vi "START1.vi"() -> ()   [LabVIEW 2024]
uses:
  <vilib>/Utility/file.llb/Read Delimited Spreadsheet (DBL).vi
panel:
  in  "stop":bool
  out "Flow Rate Display":dynamicdata(graph)
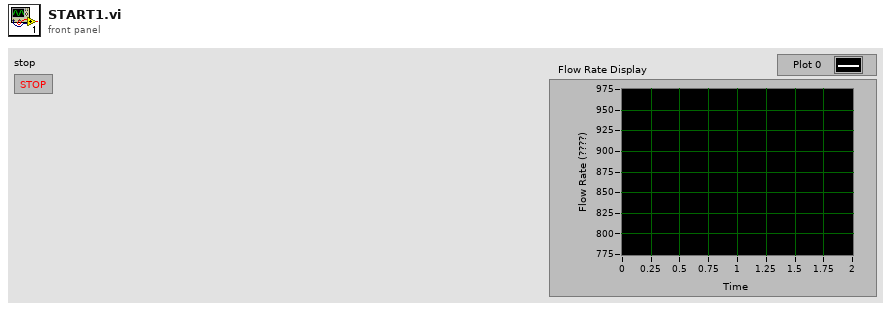
[diagram p1: front panel]
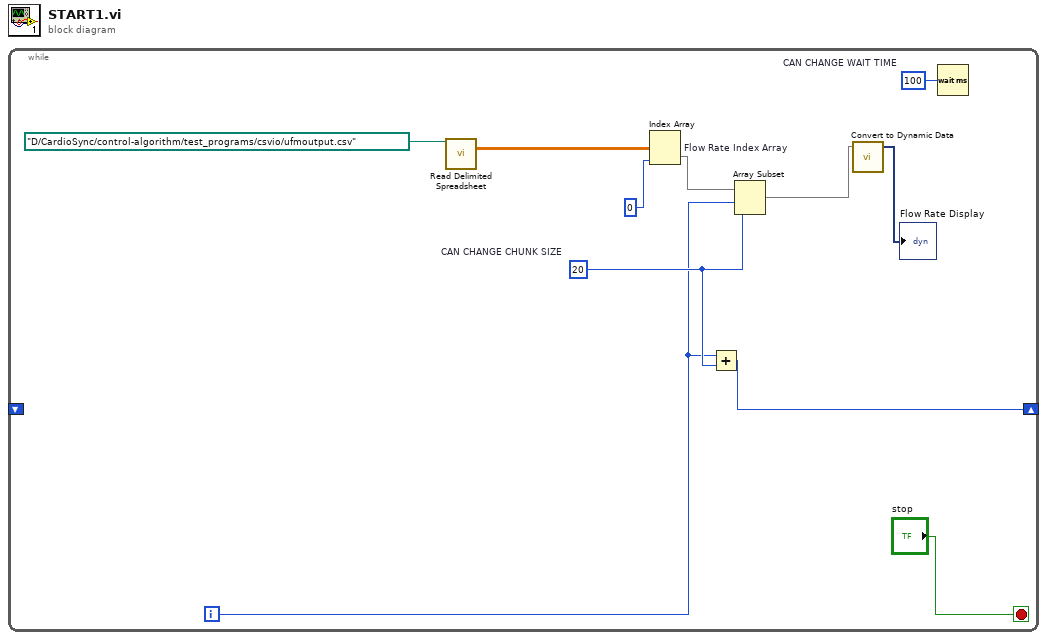
[diagram p0: block diagram]
diagram:
  n1 = while {
    shift-right: [w3] -> _
    shift-left: _ -> [_]
    i -> [w5]
    stop <- "stop" stop-if-true
    w6 = u32 100  # CAN CHANGE WAIT TIME
    w7 = 20  # CAN CHANGE CHUNK SIZE
    n2 = call-poly <vilib>:"Read Delimited Spreadsheet.vi"("file path (dialog if empty)"=path "D:/CardioSync/control-algorithm/test_programs/csvio/ufmoutput.csv") -> ("all rows"=w9:dbl[][])  [unwired: 9 in, 5 out]
    n3 = Index Array "Flow Rate Index Array"(array=w9, index (col)=0 ("disabled index (col)")) -> (element=w8:dbl[])  [unwired: 1 in]
    n4 = Add(x=w5, y=w7) -> (x+y=w3:i32)
    n5 = Array Subset(array=w8, index=w5, length=w7) -> (w1:dbl[])
    n6 = call "Convert to Dynamic Data"("Array"=w1) -> ("Dynamic Data Type"=→"Flow Rate Display":dynamicdata)  [unwired: 3 in]
    n7 = Wait (ms)(milliseconds to wait=w6) -> ()  [unwired: 1 out]
  }
